vi "newTurretLogical.vi"() -> ()   [LabVIEW 2016]
uses:
  <vilib>/Rock Robotics/WPI/MotorControl/WPI_MotorControlDeviceRef.ctl
  <vilib>/Rock Robotics/WPI/MotorControl/WPI_MotorControlType.ctl
  <vilib>/Rock Robotics/SystemInterfaces/DIO/FPGA_DIOPWMChannel.ctl
  <vilib>/Rock Robotics/WPI/PWM/WPI_PWMDeadband.ctl
  <vilib>/addons/control/pid/pid.llb/PID (DBL).vi
  <vilib>/addons/control/pid/NI_PID_pid.lvlib
panel:
  in  "turretMotorDevRef":T1={"DeviceStatus"={"status"=FALSE, "code"=0, "source"=""}, "Type"=enum."PWM", "PWM"={"PWM Channel"=enum."Invalid", "DeadBand"={"Name"="", "maxPositivePwm"=0, "minPositivePwm"=0, "centerPwm"=0, "maxNegativePwm"=0, "minNegativePwm"=0, "angularRange"=0}}, "CAN"={"Device Number"=0, "SetOutput VI Ref"=variant(enum8{"Percent VBus", "Current", "Speed", "Position", "Voltage"} enum."Percent VBus"), "GetOutput VI Ref"=variant(refnum<k1> refnum), "Enable VI Ref"=variant(dbl 12.0), "Disable VI Ref"=variant(enum8{"Percent VBus", "Speed", "Position", "Slave", "Unchanged / Invalid"} enum."Percent VBus"), "Data"=variant}, "Invert"=FALSE}
  in  "tolerance":dbl
  in  "desiredAngle":dbl format="%.2f"
  in  "evalPeriod":dbl
  out "done":bool
  in  "range":cluster{"high":dbl, "low":dbl}
  in  "softstop":dbl
  in  "currentAngle":dbl format="%.2f"
  in  "output range":cluster{"output high":dbl, "output low":dbl}={"output high"=100.0, "output low"=-100.0} {"output low" format="%.2f"; "output high" format="%.2f"}
  in  "PID gains":T5={"proportional gain (Kc)"=1.0, "integral time (Ti, min)"=0.01, "derivative time (Td, min)"=0.0} {"derivative time (Td, min)" format="%.3f"; "integral time (Ti, min)" format="%.3f"; "proportional gain (Kc)" format="%.3f"}
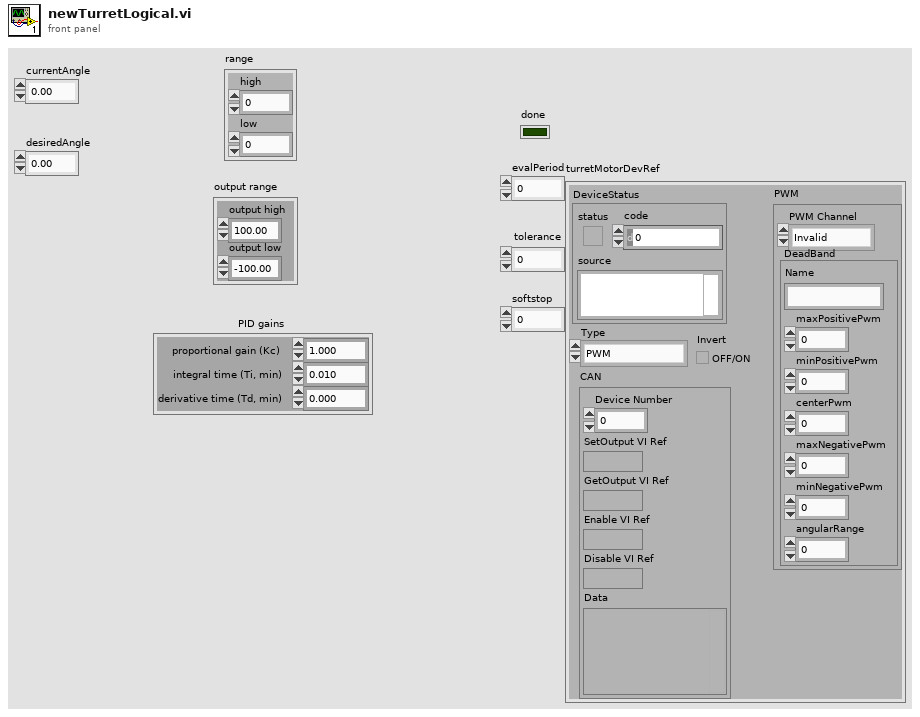
[diagram p1: front panel]
types:
  T1 = typedef "WPI_MotorControlDeviceRef.ctl" = cluster{"DeviceStatus":errorcluster, "Type":T2, "PWM":cluster{"PWM Channel":T3, "DeadBand":T4}, "CAN":cluster{"Device Number":u8, "SetOutput VI Ref":variant, "GetOutput VI Ref":variant, "Enable VI Ref":variant, "Disable VI Ref":variant, "Data":variant}, "Invert":bool}
  T2 = typedef "WPI_MotorControlType.ctl" = enum16{"PWM", "CAN"}
  T3 = typedef "FPGA_DIOPWMChannel.ctl" = enum8{"PWM 0", "PWM 1", "PWM 2", "PWM 3", "PWM 4", "PWM 5", "PWM 6", "PWM 7", "PWM 8", "PWM 9", "PWM MXP 0", "PWM MXP 1", "PWM MXP 2", "PWM MXP 3", "PWM MXP 4", "PWM MXP 5", "PWM MXP 6", "PWM MXP 7", "PWM MXP 8", "PWM MXP 9", "Invalid"}
  T4 = typedef "WPI_PWMDeadband.ctl" = cluster{"Name":string, "maxPositivePwm":i32, "minPositivePwm":i32, "centerPwm":i32, "maxNegativePwm":i32, "minNegativePwm":i32, "angularRange":u16}
  T5 = cluster{"proportional gain (Kc)":dbl, "integral time (Ti, min)":dbl, "derivative time (Td, min)":dbl}
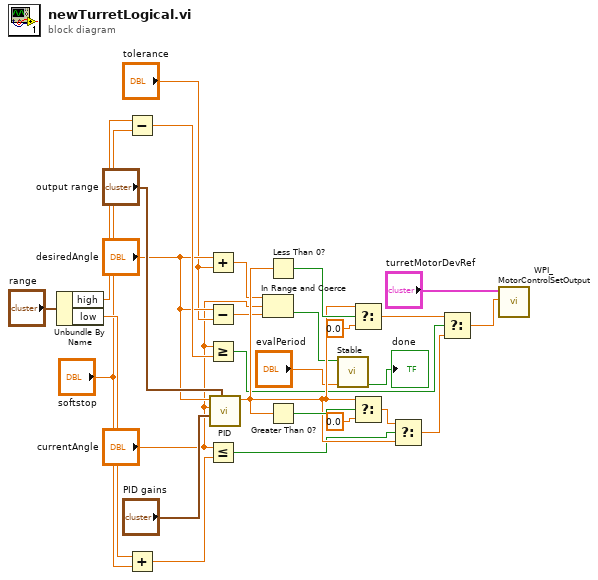
[diagram p0: block diagram]
diagram:
  n1 = Unbundle By Name("range") -> ("high"=w20:dbl, "low"=w19:dbl)
  n2 = Subtract(x=w20, y="softstop") -> (x-y=w14:dbl)
  n3 = Add(x=w19, y="softstop") -> (x+y=w12:dbl)
  n4 = Add(x="desiredAngle", y="tolerance") -> (x+y=w8:dbl)
  n5 = Subtract(x="desiredAngle", y="tolerance") -> (x-y=w7:dbl)
  n6 = Greater Or Equal?(x="currentAngle", y=w14) -> (x >= y?=w13:bool)
  n7 = Less Or Equal?(x="currentAngle", y=w12) -> (x <= y?=w11:bool)
  n8 = call-poly <vilib>:"PID.vi"("output range"="output range", "PID gains"="PID gains", "process variable"="currentAngle", "setpoint"="desiredAngle") -> ("output"=w15:dbl)  [unwired: 6 in, 1 out]
  n9 = In Range and Coerce(upper limit=w8, x="currentAngle", lower limit=w7) -> (In Range?=w6:bool)  [unwired: 1 out]
  n10 = Less Than 0?(x=w15) -> (x < 0?=w17:bool)
  n11 = Greater Than 0?(x=w15) -> (x > 0?=w16:bool)
  n12 = call <userlib>:"Stable.vi"("Eval Period (sec)"="evalPeriod", "Signal Input"=w6) -> ("Stable"=→"done":bool)  [unwired: 9 in]
  n13 = Select(t=w15, s=w17, f=0.0) -> (s? t:f=w24:dbl)
  n14 = Select(t=w15, s=w16, f=0.0) -> (s? t:f=w23:dbl)
  n15 = Select(t=w23, s=w11, f=w15) -> (s? t:f=w25:dbl)
  n16 = Select(t=w24, s=w13, f=w25) -> (s? t:f=w2:dbl)
  n17 = call <vilib>:"WPI_MotorControlSetOutput.vi"("Output"=w2, "MotorControlDevRef"="turretMotorDevRef") -> ()  [unwired: 7 in, 3 out]
